vi "Bench.vi"() -> ()   [LabVIEW 2026]
panel:
  out "elapsed ms":dbl
  out "reply":string
  in  "command":string
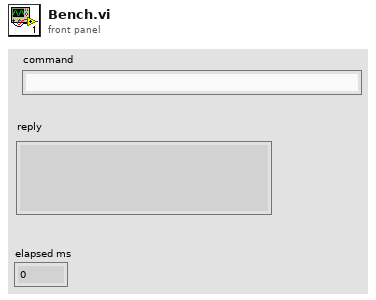
[diagram p1: front panel]
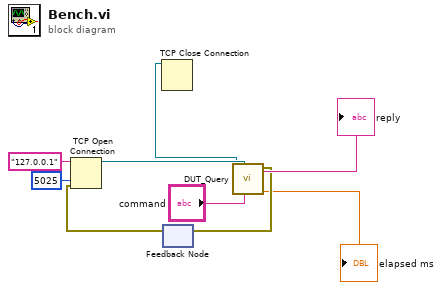
[diagram p0: block diagram]
diagram:
  n1 = feedback #1() -> (w3:errorcluster)  [unwired: 1 in]
  n2 = TCP Open Connection(address="127.0.0.1", remote port or service name=u16 5025, error in (no error)=w3) -> (connection ID=w7:refnum<k5>)  [unwired: 2 in, 1 out]
  n3 = call "DUT_Query.vi"("command"="command", "connection ID"=w7) -> ("error out"=w4:errorcluster, "reply"=→"reply":string, "elapsed ms"=→"elapsed ms":dbl, "connection ID out"=w2:refnum<k5>)  [unwired: 6 in]
  n4 = TCP Close Connection(connection ID=w2) -> ()  [unwired: 2 in, 2 out]
  n5 = feedback-in #1(w4) -> ()
